vi "Write setup configuration.vi"(8 "error in (no error)":errorcluster, 11 "Channel in":refnum<class "Channel.lvclass">) -> (0 "error out":errorcluster, 3 "Channel out":refnum<class "Channel.lvclass">)   [LabVIEW 2018, in "Channel.lvclass"]
uses:
  Channel.lvclass
  Channel.lvclass/Channel.ctl
  Simulated_CCD_Camera/Simulated Camera.lvclass
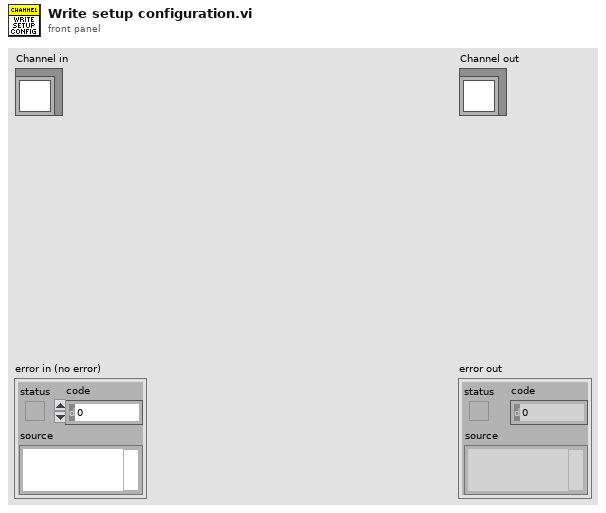
[diagram p1: front panel]
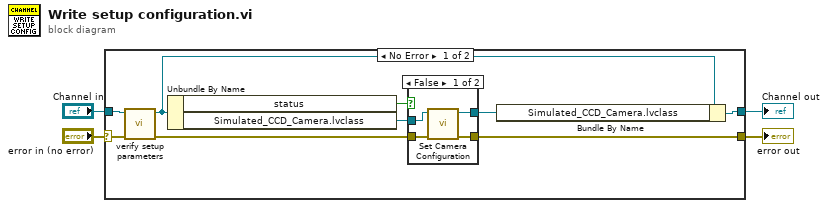
[diagram p0: block diagram]
diagram:
  n1 = case shown="No Error" "error in (no error)" {
    selector: "error in (no error)" -> [w8 w21]
    tunnel: [w12 w21] -> w3
    tunnel: [w10 w20] -> w1
    tunnel: "Channel in" -> [w9 w20]
    frame No Error {
      n2 = call "verify setup parameters.vi"("error in (no error)"=w8, "Channel in"=w9) -> ("error out"=w5:errorcluster, "Channel out"=w6:refnum<class "Channel.lvclass">)  [unwired: 8 in]
      n3 = Unbundle By Name(w6) -> ("status"=w7:bool, "Simulated_CCD_Camera.lvclass"=w13:refnum<class "Simulated Camera.lvclass">)
      n4 = case shown="False" w7 {
        tunnel: w13 -> [w17 w19]
        tunnel: w5 -> [w16 w18]
        tunnel: [w14 w18] -> w12
        tunnel: [w15 w19] -> w11
        frame False {
          n5 = call-dynamic "Set Camera Configuration.vi"("error in (no error)"=w16, "CCDCamera in"=w17) -> ("error out"=w14:errorcluster, "CCDCamera out"=w15:refnum<class "Simulated Camera.lvclass">)  [unwired: 8 in]
        }
        frame True {
        }
      }
      n6 = Bundle By Name(cluster=w6, "Simulated_CCD_Camera.lvclass"=w11) -> (w10:refnum<class "Channel.lvclass">)
    }
    frame Error {
    }
  }
  "error out" <- w3
  "Channel out" <- w1
